vi "Set Comparison String.vi"(4 "Report Text 2":string="ProgramNumber=1\nProgramDefined=YES\nProgramDisabled=NO\nProgramName=Ramping01\\00\\00\\00\\00\\00\\00\\00\nProgramFreqTable[00]Allowed=NO\nProgramFreqTable[01]Allowed=NO\nProgramFreqTable[02]Allowed=NO\nProgramFreqTable[03]Allowed=NO\nProgramFreqTable[04]Allowed=NO\nProgramFreqTable[05]Allowed=NO\nProgramFreqTable[06]Allowed=NO\nProgramFreqTable[07]Allowed=NO\nProgramFreqTable[08]Allowed=NO\nProgramFreqTable[09]Allowed=NO\nProgramFreqTable[10]Allowed=NO\nProgramFreqTable[11]Allowed=NO\nProgramFreqTable[12]Allowed=NO\nProgramFreqTable[13]Allowed=NO\nProgramFreqTable[14]Allowed=NO\nProgramFreqTable[15]Allowed=NO\nProgramFreqTable[16]Allowed=NO\nProgramFreqTable[17]Allowed=NO\nProgramFreqTable[18]Allowed=NO\nProgramFreqTable[19]Allowed=NO\nProgramFreqTable[20]Allowed=NO\nProgramFreqTable[21]Allowed=NO\nProgramFreqTable[22]Allowed=YES\nProgramFreqTable[23]Allowed=NO\nProgramFreqTable[24]Allowed=NO\nProgramFreqTable[25]Allowed=NO\nProgramFreqTable[26]Allowed=NO\nProgramFreqTable[27]Allowed=NO\nProgramFreqTable[28]Allowed=NO\nProgramFreqTable[29]Allowed=NO\nProgramFreqTable[30]Allowed=NO\nProgramFreqTable[31]Allowed=NO\nProgramFreqTable[32]Allowed=NO\nProgramFreqTable[33]Allowed=NO\nProgramFreqTable[34]Allowed=NO\nProgramFreqTable[35]Allowed=NO\nProgramFreqTable[36]Allowed=NO\nProgramFreqTable[37]Allowed=NO\nProgramFreqTable[38]Allowed=NO\nProgramFreqTable[39]Allowed=NO\nProgramFreqTable[40]Allowed=NO\nProgramFreqTable[41]Allowed=NO\nProgramFreqTable[42]Allowed=NO\nProgramFreqTable[43]Allowed=NO\nProgramFreqTable[44]Allowed=NO\nProgramFreqTable[45]Allowed=NO\nProgramFreqTable[46]Allowed=NO\nProgramFreqTable[47]Allowed=NO\nProgramFreqTable[48]Allowed=NO\nProgramFreqTable[49]Allowed=NO\nProgramFreqTable[50]Allowed=NO\nProgramFreqTable[51]Allowed=NO\nProgramFreqTable[52]Allowed=NO\nProgramFreqTable[53]Allowed=NO\nProgramFreqTable[54]Allowed=NO\nProgramFreqTable[55]Allowed=NO\nProgramFreqTable[56]Allowed=NO\nProgramFreqTable[57]Allowed=NO\nProgramFreqTable[58]Allowed=NO\nProgramFreqTable[59]Allowed=NO\nProgramFreqTable[60]Allowed=NO\nProgramFreqTable[61]Allowed=NO\nProgramFreqTable[62]Allowed=NO\nProgramFreqTable[63]Allowed=NO\nProgramFrequencyIndex=22\nPA_Defined=YES\nPB_Defined=YES\nPC_Defined=YES\nPD_Defined=YES\n\n-- PULSE PA --\nPulseNamePA=P1\\00\\00\\00\\00\\00\\00\\00\\00\\00\\00\\00\\00\\00\\00\nAmplitudeLowLimitPA=10005\nAmplitudeStepPA=20\nAmplitudeStepIndexPA=1\nPulseWidthLowLimitPA=200\nPulseWidthHighLimitPA=1000\nPulseWidthPA=500\nElectrodeAmpPercentPA[CH01]=0\nElectrodeAmpPercentPA[CH02]=0\nElectrodeAmpPercentPA[CH03]=0\nElectrodeAmpPercentPA[CH04]=0\nElectrodeAmpPercentPA[CH05]=0\nElectrodeAmpPercentPA[CH06]=0\nElectrodeAmpPercentPA[CH07]=0\nElectrodeAmpPercentPA[CH08]=0\nElectrodeAmpPercentPA[CH09]=0\nElectrodeAmpPercentPA[CH10]=0\nElectrodeAmpPercentPA[CH11]=0\nElectrodeAmpPercentPA[CH12]=0\nElectrodeAmpPercentPA[CH13]=0\nElectrodeAmpPercentPA[CH14]=0\nElectrodeAmpPercentPA[CH15]=0\nElectrodeAmpPercentPA[CH16]=0\nElectrodeAmpPercentPA[CH17]=0\nElectrodeAmpPercentPA[CH18]=0\nElectrodeAmpPercentPA[CH19]=0\nElectrodeAmpPercentPA[CH20]=0\nElectrodeAmpPercentPA[CH21]=0\nElectrodeAmpPercentPA[CH22]=0\nElectrodeAmpPercentPA[CH23]=0\nElectrodeAmpPercentPA[CH24]=0\nElectrodeAmpPercentPA[CH25]=-100\nElectrodeAmpPercentPA[CH26]=100\n\n-- PULSE PB --\nPulseNamePB=P2\\00\\00\\00\\00\\00\\00\\00\\00\\00\\00\\00\\00\\00\\00\nAmplitudeLowLimitPB=8010\nAmplitudeStepPB=20\nAmplitudeStepIndexPB=1\nPulseWidthLowLimitPB=200\nPulseWidthHighLimitPB=1000\nPulseWidthPB=600\nElectrodeAmpPercentPB[CH01]=0\nElectrodeAmpPercentPB[CH02]=0\nElectrodeAmpPercentPB[CH03]=0\nElectrodeAmpPercentPB[CH04]=0\nElectrodeAmpPercentPB[CH05]=0\nElectrodeAmpPercentPB[CH06]=0\nElectrodeAmpPercentPB[CH07]=0\nElectrodeAmpPercentPB[CH08]=0\nElectrodeAmpPercentPB[CH09]=0\nElectrodeAmpPercentPB[CH10]=0\nElectrodeAmpPercentPB[CH11]=0\nElectrodeAmpPercentPB[CH12]=0\nElectrodeAmpPercentPB[CH13]=0\nElectrodeAmpPercentPB[CH14]=0\nElectrodeAmpPercentPB[CH15]=0\nElectrodeAmpPercentPB[CH16]=0\nElectrodeAmpPercentPB[CH17]=0\nElectrodeAmpPercentPB[CH18]=0\nElectrodeAmpPercentPB[CH19]=0\nElectrodeAmpPercentPB[CH20]=0\nElectrodeAmpPercentPB[CH21]=0\nElectrodeAmpPercentPB[CH22]=0\nElectrodeAmpPercentPB[CH23]=0\nElectrodeAmpPercentPB[CH24]=0\nElectrodeAmpPercentPB[CH25]=-100\nElectrodeAmpPercentPB[CH26]=100\n\n-- PULSE PC --\nPulseNamePC=P3\\00\\00\\00\\00\\00\\00\\00\\00\\00\\00\\00\\00\\00\\00\nAmplitudeLowLimitPC=5010\nAmplitudeStepPC=20\nAmplitudeStepIndexPC=1\nPulseWidthLowLimitPC=200\nPulseWidthHighLimitPC=1000\nPulseWidthPC=700\nElectrodeAmpPercentPC[CH01]=0\nElectrodeAmpPercentPC[CH02]=0\nElectrodeAmpPercentPC[CH03]=0\nElectrodeAmpPercentPC[CH04]=0\nElectrodeAmpPercentPC[CH05]=0\nElectrodeAmpPercentPC[CH06]=0\nElectrodeAmpPercentPC[CH07]=0\nElectrodeAmpPercentPC[CH08]=0\nElectrodeAmpPercentPC[CH09]=0\nElectrodeAmpPercentPC[CH10]=0\nElectrodeAmpPercentPC[CH11]=0\nElectrodeAmpPercentPC[CH12]=0\nElectrodeAmpPercentPC[CH13]=0\nElectrodeAmpPercentPC[CH14]=0\nElectrodeAmpPercentPC[CH15]=0\nElectrodeAmpPercentPC[CH16]=0\nElectrodeAmpPercentPC[CH17]=0\nElectrodeAmpPercentPC[CH18]=0\nElectrodeAmpPercentPC[CH19]=0\nElectrodeAmpPercentPC[CH20]=0\nElectrodeAmpPercentPC[CH21]=0\nElectrodeAmpPercentPC[CH22]=0\nElectrodeAmpPercentPC[CH23]=0\nElectrodeAmpPercentPC[CH24]=0\nElectrodeAmpPercentPC[CH25]=-100\nElectrodeAmpPercentPC[CH26]=100\n\n-- PULSE PD --\nPulseNamePD=P4\\00\\00\\00\\00\\00\\00\\00\\00\\00\\00\\00\\00\\00\\00\nAmplitudeLowLimitPD=2010\nAmplitudeStepPD=20\nAmplitudeStepIndexPD=1\nPulseWidthLowLimitPD=200\nPulseWidthHighLimitPD=1000\nPulseWidthPD=800\nElectrodeAmpPercentPD[CH01]=0\nElectrodeAmpPercentPD[CH02]=0\nElectrodeAmpPercentPD[CH03]=0\nElectrodeAmpPercentPD[CH04]=0\nElectrodeAmpPercentPD[CH05]=0\nElectrodeAmpPercentPD[CH06]=0\nElectrodeAmpPercentPD[CH07]=0\nElectrodeAmpPercentPD[CH08]=0\nElectrodeAmpPercentPD[CH09]=0\nElectrodeAmpPercentPD[CH10]=0\nElectrodeAmpPercentPD[CH11]=0\nElectrodeAmpPercentPD[CH12]=0\nElectrodeAmpPercentPD[CH13]=0\nElectrodeAmpPercentPD[CH14]=0\nElectrodeAmpPercentPD[CH15]=0\nElectrodeAmpPercentPD[CH16]=0\nElectrodeAmpPercentPD[CH17]=0\nElectrodeAmpPercentPD[CH18]=0\nElectrodeAmpPercentPD[CH19]=0\nElectrodeAmpPercentPD[CH20]=0\nElectrodeAmpPercentPD[CH21]=0\nElectrodeAmpPercentPD[CH22]=0\nElectrodeAmpPercentPD[CH23]=0\nElectrodeAmpPercentPD[CH24]=0\nElectrodeAmpPercentPD[CH25]=-100\nElectrodeAmpPercentPD[CH26]=100", 5 "Sequence Context":refnum<k7>) -> (0 "error out":errorcluster, 2 "Report Text":string)   [LabVIEW 2010]
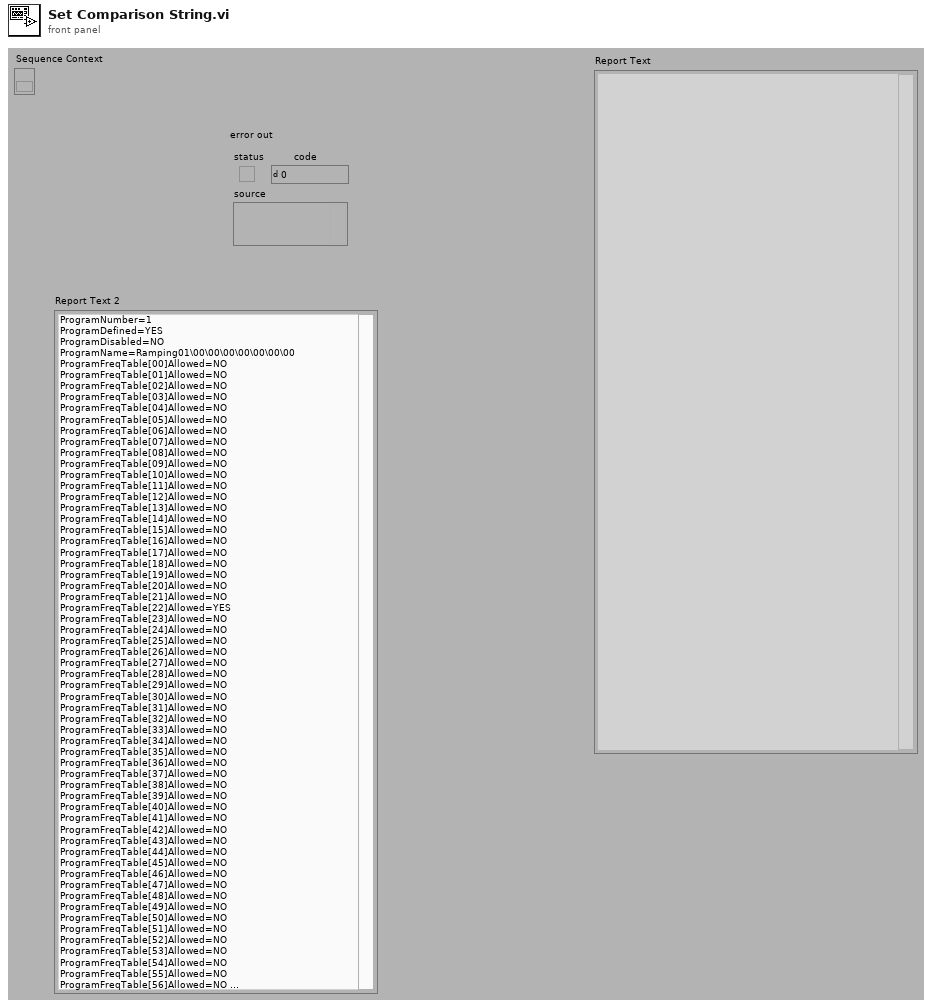
[diagram p1: front panel]
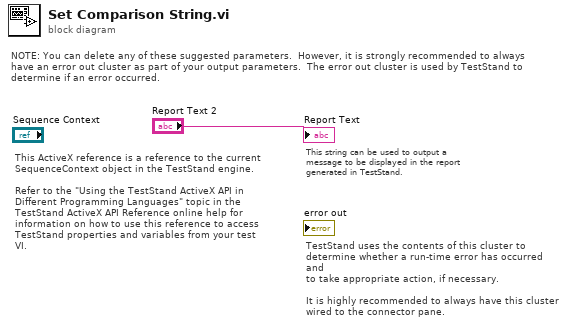
[diagram p0: block diagram]
diagram:
  # "TestStand uses the contents of this cluster to\ndetermine whether a run-time error has occurred and\nto take appropriate action, if necessary.\n\nIt is highly recommended to always have this cluster\nwired to the connector pane."
  # "This string can be used to output a\nmessage to be displayed in the report\ngenerated in TestStand."
  # "NOTE: You can delete any of these suggested parameters.  However, it is strongly recommended to always have an error out cluster as part of your output parameters.  The error out cluster is used by TestStand to determine if an error occurred."
  # "This ActiveX reference is a reference to the current\nSequenceContext object in the TestStand engine.\n\nRefer to the \"Using the TestStand ActiveX API in\nDifferent Programming Languages\" topic in the \nTestStand ActiveX API Reference online help for\ninformation on how to use this reference to access\nTestStand properties and variables from your test VI."
  "Report Text" <- "Report Text 2"
